vi "Configure Output.vi"(0 "reference in":refnum<class "BKP-911x Power Supply.lvclass">, 2 "Enable Output (T: Enable)":bool=TRUE, 5 "error in (no error)":errorcluster) -> (14 "reference out":refnum<class "BKP-911x Power Supply.lvclass">, 19 "error out":errorcluster)   [LabVIEW 2018, in "BKP-911x Power Supply.lvclass"]
uses:
  BKP-911x Power Supply.lvclass
  <instrlib>/BK Precision 911X Series/BK Precision 911X Series.lvlib
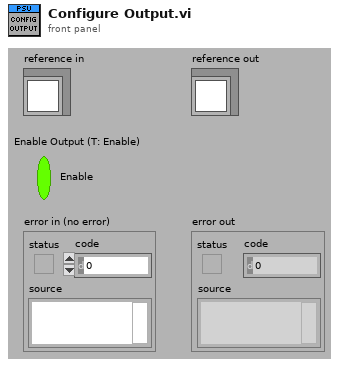
[diagram p1: front panel]
types:
  T1 = typedef "BKP-911x Power Supply.lvclass/ObjectAttributes.ctl" = cluster{"VISA resource name":refnum<visa-resource-name>, "Simulated?":bool, "Latest Values":dbl[], "Signal List":T2[], "Voltage Setpoint (V)":dbl, "Current Limit (A)":dbl, "Output Enabled?":bool}
  T2 = typedef "IO Signal List.ctl" = enum16{"Timestamp", "PSU_FB_U_VDC", "PSU_FB_I_AMP", "PSU_FB_W_WATT", "PSU_CMD_U_VDC", "PSU_CMD_I_AMP", "PSU_CMD_OUTPUT", "LCR_PRIMARY", "LCR_SECONDARY", "UV_R_Ohm", "UW_R_Ohm", "VW_R_Ohm", "UV_L_H", "UW_L_H", "VW_L_H", "U_U_VDC", "V_U_VDC", "W_U_VDC", "U_I_AMP", "V_I_AMP", "W_I_AMP", "PWM_CMD_DC_%", "PWM_CMD_VDC", "PWM_CMD_Hz", "PWM_FB_DC_%", "PWM_FB_VDC", "PWM_FB_Hz", "DO_RELAY_U_LCR_A", "DO_RELAY_V_LCR_A", "DO_RELAY_V_LCR_B", "DO_RELAY_W_LCR_B", "DIFF_UV_UW_L_H", "DIFF_UV_VW_L_H", "DIFF_UW_VW_L_H", "DIFF_UV_UW_R_Ohm", "DIFF_UV_VW_R_Ohm", "DIFF_UW_VW_R_Ohm", "DIFF_UV_U_VDC", "DIFF_UW_U_VDC", "DIFF_VW_U_VDC"}
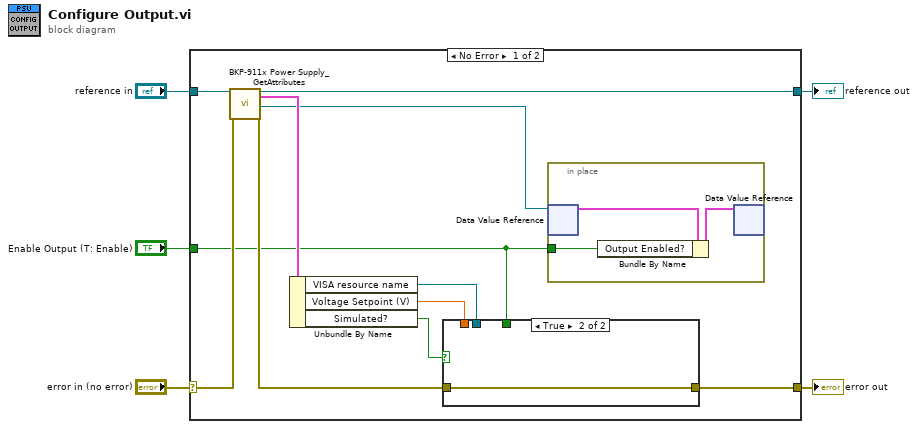
[diagram p0: block diagram]
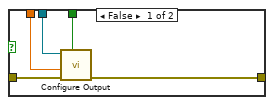
[diagram p2: hidden frame]
diagram:
  n1 = case shown="No Error" "error in (no error)" {
    selector: "error in (no error)" -> [w16 w27]
    tunnel: [w11 w27] -> w4
    tunnel: [w13 w26] -> w2
    tunnel: "reference in" -> [w14 w26]
    tunnel: "Enable Output (T: Enable)" -> [w7 _]
    frame No Error {
      n2 = call "BKP-911x Power Supply_GetAttributes.vi"("reference in"=w14, "error in (no error)"=w16) -> ("reference out"=w13:refnum<class "BKP-911x Power Supply.lvclass">, "Data"=w15:T1, "DataRef"=w8:refnum<data-value>, "error out"=w12:errorcluster)  [unwired: 14 in]
      n3 = Unbundle By Name(w15) -> ("VISA resource name"=w10:refnum<visa-resource-name>, "Voltage Setpoint (V)"=w9:dbl, "Simulated?"=w6:bool)
      n4 = case shown="True" w6 {
        tunnel: w12 -> [w21 w22]
        tunnel: [w20 w22] -> w11
        tunnel: w10 -> [w19 _]
        tunnel: w9 -> [w18 _]
        tunnel: w7 -> [w17 _]
        frame False {
          n5 = call <instrlib>:"Configure Output.vi"("Enable Output (T: Enable)"=w17, "error in (no error)"=w21, "Voltage Level (0.0 V)"=w18, "VISA resource name"=w19) -> ("error out"=w20:errorcluster)  [unwired: 6 in, 1 out]
        }
        frame True {
        }
      }
      n6 = in-place {
        in-place-border: w7 -> [w24]
        n7 = in-place-dvr #1(w8) -> (w25:T1)  [unwired: 1 out]
        n8 = Bundle By Name(cluster=w25, "Output Enabled?"=w24) -> (w23:T1)
        n9 = in-place-dvr #1(w23) -> ()  [unwired: 2 out]
      }
    }
    frame Error {
    }
  }
  "error out" <- w4
  "reference out" <- w2
